vi "WriteControlSettings.vi"(8 "error in (no error)":errorcluster, 11 "VI Refnum":refnum<vi>) -> (0 "error out":errorcluster)   [LabVIEW 2013, in "main.lvlib"]
uses:
  main.lvlib
  <vilib>/Utility/config.llb/NI_LVConfig.lvlib
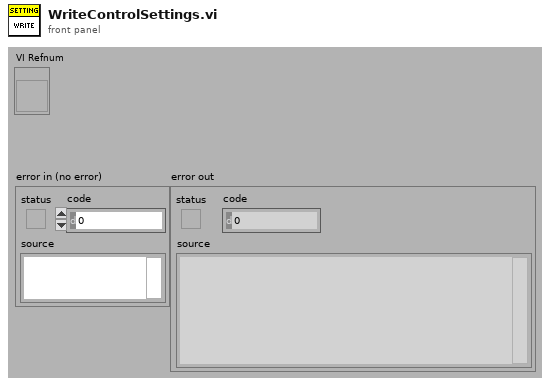
[diagram p1: front panel]
types:
  T1 = typedef "NI_LVConfig.lvlib/Config Data RefNum.ctl" = refnum<k1>
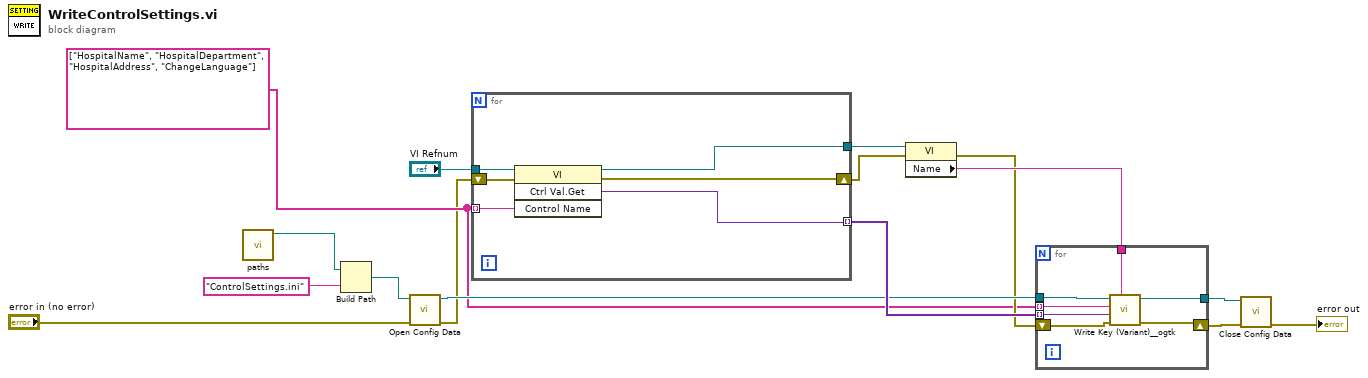
[diagram p0: block diagram]
diagram:
  w7 = string[] ["HospitalName", "HospitalDepartment", "HospitalAddress", "ChangeLanguage"]
  n1 = call "paths.vi"() -> ("PubAppData"=w6:path)  [unwired: 8 in, 3 out]
  n2 = Build Path(base path=w6, name or relative path="ControlSettings.ini") -> (appended path=w13:path)
  n3 = call <vilib>:"Open Config Data.vi"("error in (no error)"="error in (no error)", "configuration file path"=w13) -> ("error out"=w5:errorcluster, "refnum"=w10:T1)  [unwired: 7 in, 1 out]
  n4 = for {
    tunnel: "VI Refnum" -> [w22]
    tunnel: w7 -> [w18] mode=indexing
    tunnel: [w21] -> w14
    shift-right: [w20] -> w9
    shift-left: w5 -> [w19]
    tunnel: [w17] -> w12 mode=indexing
    n5 = invoke class="VI" method="Ctrl Val.Get"(reference=w22, error in=w19, "Control Name"=w18) -> (reference out=w21:refnum<vi>, error out=w20:errorcluster, "Get Control Value Variant"=w17:variant)  [unwired: 1 in, 1 out]
  }
  n6 = property class="VI"(reference=w14, error in=w9) -> (error out=w8:errorcluster, "Name"=w11:string)  [unwired: 1 out]
  n7 = for {
    tunnel: w12 -> [w28] mode=indexing
    tunnel: w7 -> [w27] mode=indexing
    tunnel: w11 -> [w26]
    tunnel: w10 -> [w25]
    shift-right: [w29] -> w2
    shift-left: w8 -> [w24]
    tunnel: [w23] -> w3
    n8 = call <userlib>:"Write Key (Variant)__ogtk.vi"("section"=w26, "error in (no error)"=w24, "key-value"=w28, "key (optional)"=w27, "refnum"=w25) -> ("error out"=w29:errorcluster, "refnum out"=w23:T1)  [unwired: 5 in]
  }
  n9 = call <vilib>:"Close Config Data.vi"("error in (no error)"=w2, "refnum"=w3) -> ("error out"=→"error out":errorcluster)  [unwired: 8 in, 1 out]
